vi "loop_time.vi"(0 "previous timer value":u32) -> (1 "millisecond timer value":u32, 2 "Loop Time [ms]":u32)   [LabVIEW 2022 SP3]
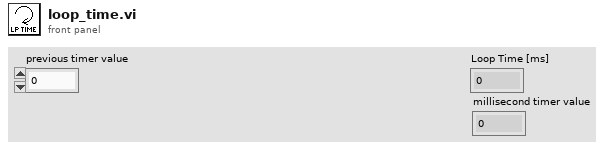
[diagram p1: front panel]
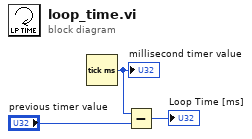
[diagram p0: block diagram]
diagram:
  n1 = Tick Count (ms)() -> (millisecond timer value=w3:u32)
  "millisecond timer value" <- w3
  n2 = Subtract(x=w3, y="previous timer value") -> (x-y=→"Loop Time [ms]":u32)
